vi "Run Test.vi"(8 "error in (no error)":errorcluster, 11 "LED Board Visual Test in":refnum<class "LED Board Setup.lvclass">) -> (0 "error out":errorcluster, 1 "Positions":i32[](array[numeric]), 2 "Tests Passed":bool[](array[boolean]), 3 "LED Board Visual Test out":refnum<class "LED Board Setup.lvclass">, 5 "Fail Codes":string[](array[string]))   [LabVIEW 2015, in "LED Board Setup.lvclass"]
uses:
  LED Board Setup.lvclass
  CBTF Applications/LED Board Testing/Main/Application/Application/Class/typedefs/Instrument Selector -- Enum.ctl
  Classes/Instruments/DC Power Supply/DC Power Supply/Class/DC Power Supply.lvclass
  Test Class/Test Class.lvclass
  CBTF Applications/LED Board Testing/Main/Application/Application/Class/LED Board.lvclass
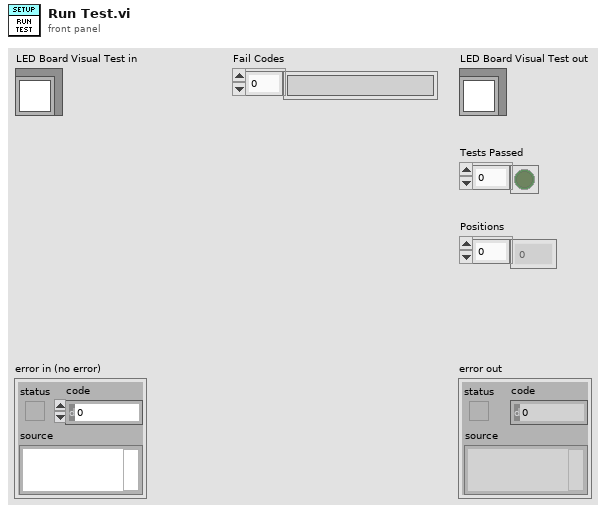
[diagram p1: front panel]
types:
  T1 = typedef "LED Board.lvlib/LED Board.lvclass/Instrument Selector -- Enum.ctl" = enum16{"DC Power Supply 1", "DC Power Supply 2", "DC Power Supply 3", "Camera", "Switch Executive"}
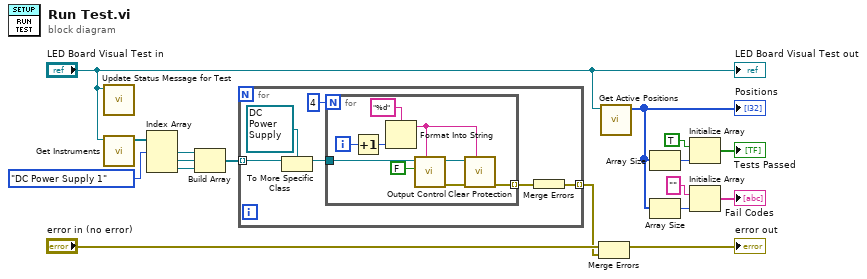
[diagram p0: block diagram]
diagram:
  n1 = call-dynamic "Update Status Message for Test.vi"("LED Board Power Test in"="LED Board Visual Test in") -> ()  [unwired: 11 in]
  n2 = call "Get Instruments.vi"("Test Class in"="LED Board Visual Test in") -> ("Instruments"=w10:refnum<class "Instrument.lvclass">[])  [unwired: 9 in, 1 out]
  n3 = Index Array(array=w10, index #1=Instrument_Selector_--_Enum."DC Power Supply 1" ("Instrument")) -> (element #1=w8:refnum<class "Instrument.lvclass">, element #2=w7:refnum<class "Instrument.lvclass">, element #3=w6:refnum<class "Instrument.lvclass">)  [unwired: 2 in]
  n4 = Build Array(w8, w7, w6) -> (w5:refnum<class "Instrument.lvclass">[])
  n5 = for {
    tunnel: w5 -> [w23] mode=indexing
    tunnel: [w18] -> w3 mode=indexing
    n6 = To More Specific Class(target class=refnum<class "DC Power Supply.lvclass"> refnum ("DC Power Supply.lvlib:DC Power Supply.lvclass"), reference=w23) -> (specific class reference=w21:refnum<class "DC Power Supply.lvclass">)  [unwired: 1 in, 1 out]
    n7 = for {
      N: 4 -> [_]
      tunnel: w21 -> [w32]
      tunnel: [w24] -> w19 mode=indexing
      i -> [w28]
      n8 = Increment(x=w28) -> (x+1=w27:i32)
      n9 = Format Into String(format string="%d", w27) -> (resulting string=w26:string)  [unwired: 2 in, 1 out]
      n10 = call-dynamic "Output Control.vi"("Channel (\"1\")"=w26, "Enabled"=FALSE, "Acrobat Template in"=w32) -> ("error out"=w29:errorcluster, "Acrobat Template out"=w30:refnum<class "DC Power Supply.lvclass">)  [unwired: 7 in]
      n11 = call-dynamic "Clear Protection.vi"("Channel (\"1\")"=w26, "error in (no error)"=w29, "Acrobat Template in"=w30) -> ("error out"=w24:errorcluster)  [unwired: 7 in, 1 out]
    }
    n12 = Merge Errors(w19) -> (w18:errorcluster)
  }
  n13 = Merge Errors("error in (no error)", w3) -> (→"error out":errorcluster)
  n14 = call "Get Active Positions.vi"("Test Class in"="LED Board Visual Test in") -> ("Active Positions"=w13:u32[])  [unwired: 9 in, 1 out]
  "Positions" <- w13
  n15 = Array Size(array=w13) -> (size(s)=w17:i32)
  n16 = Array Size(array=w13) -> (size(s)=w14:i32)
  n17 = Initialize Array(TRUE, w17) -> (→"Tests Passed":bool[])
  n18 = Initialize Array("", w14) -> (→"Fail Codes":string[])
  "LED Board Visual Test out" <- "LED Board Visual Test in"
